vi "mod_Compute FSK samples per symbol.vi"(0 "Symbol Rate":dbl format="%.2f", 5 "Deviation (Hz)":dbl format="%.2f", 9 "Filter parameter":dbl=0.5 format="%.2f", 11 "error in (no error)":errorcluster) -> (4 "FSK samples per symbol":i32, 15 "error out":errorcluster)   [LabVIEW 2020, in "niDMT.lvlib"]
uses:
  <vilib>/addons/Modulation/niDMT.lvlib
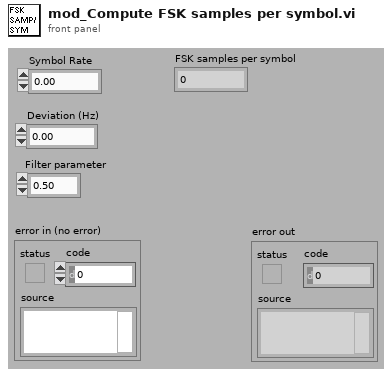
[diagram p1: front panel]
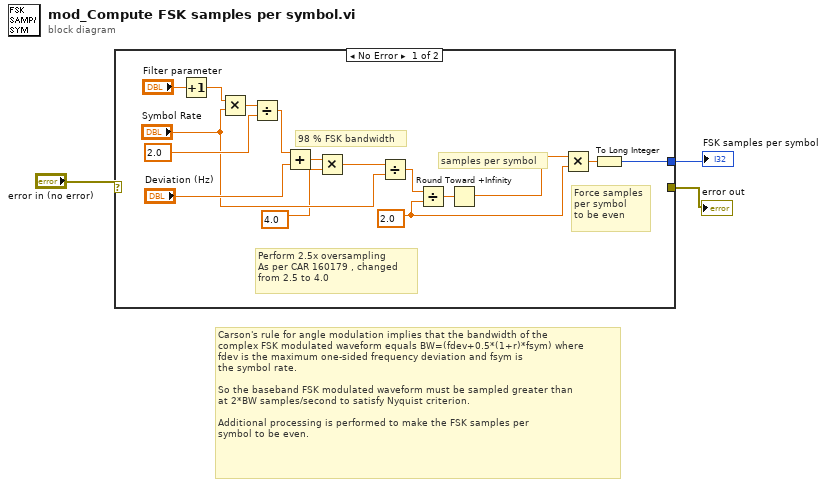
[diagram p0: block diagram]
diagram:
  # "Carson's rule for angle modulation implies that the bandwidth of the\ncomplex FSK modulated waveform equals BW=(fdev+0.5*(1+r)*fsym) where\nfdev is the maximum one-sided frequency deviation and fsym is\nthe symbol rate.\n\nSo the baseband FSK modulated waveform must be sampled greater than\nat 2*BW samples/second to satisfy Nyquist criterion.\n\nAdditional processing is performed to make the FSK samples per\nsymbol to be even."
  n1 = case shown="No Error" "error in (no error)" {
    selector: "error in (no error)" -> [_ w20]
    tunnel: [w12 _] -> w3
    tunnel: [_ w20] -> w1
    frame No Error {
      w4 = 2.0 ("y")
      # "samples per symbol"
      # "Perform 2.5x oversampling\nAs per CAR 160179 , changed\nfrom 2.5 to 4.0"
      # "98 % FSK bandwidth"
      # "Force samples\nper symbol\nto be even"
      n2 = Increment(x="Filter parameter") -> (x+1=w10:dbl)
      n3 = Multiply(x=w10, y="Symbol Rate") -> (x*y=w9:dbl)
      n4 = Divide(x=w9, y=2.0) -> (x/y=w7:dbl)
      n5 = Add(x=w7, y="Deviation (Hz)") -> (x+y=w14:dbl)
      n6 = Multiply(x=w14, y=4.0) -> (x*y=w13:dbl)
      n7 = Divide(x=w13, y="Symbol Rate") -> (x/y=w18:dbl)
      n8 = Divide(x=w18, y=w4) -> (x/y=w17:dbl)
      n9 = Round Toward +Infinity(x=w17) -> (ceil(x): smallest int >= x=w16:dbl)
      n10 = Multiply(x=w16, y=w4) -> (x*y=w15:dbl)
      n11 = To Long Integer(number=w15) -> (32bit integer=w12:i32)
    }
    frame Error {
    }
  }
  "error out" <- w1
  "FSK samples per symbol" <- w3
